vi "Query Frequency Mode.vi"(8 "error in (no error)":errorcluster, 11 "VISA resource name":refnum<visa-resource-name>) -> (0 "error out":errorcluster, 2 "Frequency Mode":T1(ring), 3 "VISA resource name out":refnum<visa-resource-name>)   [LabVIEW 2017, in "Agilent PSG MXG Series.lvlib"]
uses:
  Agilent PSG MXG Series.lvlib
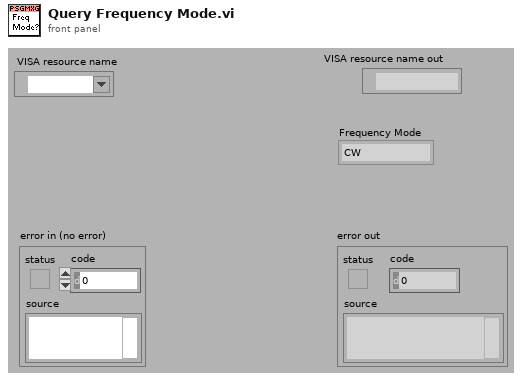
[diagram p1: front panel]
types:
  T1 = enum16{"CW", "Fixed", "Stepped Sweep", "List Sweep"}
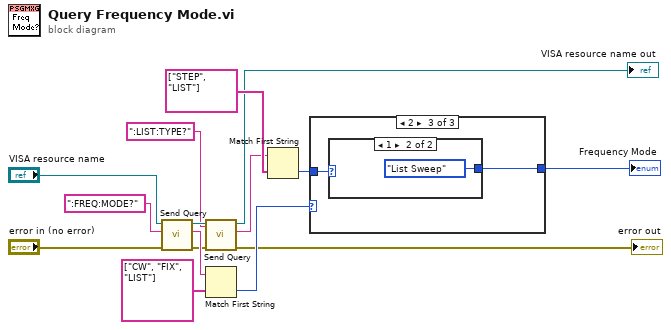
[diagram p0: block diagram]
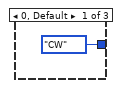
[diagram p2: hidden frame]
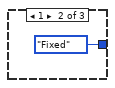
[diagram p3: hidden frame]
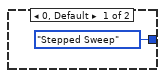
[diagram p4: hidden frame]
diagram:
  n1 = call "Send Query.vi"("error in (no error)"="error in (no error)", "write buffer"=":FREQ:MODE?", "VISA resource name"="VISA resource name") -> ("error out"=w7:errorcluster, "read buffer"=w10:string, "VISA resource name out"=w9:refnum<visa-resource-name>)  [unwired: 6 out]
  n2 = call "Send Query.vi"("error in (no error)"=w7, "write buffer"=":LIST:TYPE?", "VISA resource name"=w9) -> ("error out"=→"error out":errorcluster, "read buffer"=w6:string, "VISA resource name out"=→"VISA resource name out":refnum<visa-resource-name>)  [unwired: 6 out]
  n3 = Match First String(2:string[] ["CW", "FIX", "LIST"], 3:w10) -> (0:w5:i32)  [unwired: 1 out]
  n4 = Match First String(2:string[] ["STEP", "LIST"], 3:w6) -> (0:w3:i32)  [unwired: 1 out]
  n5 = case shown="2" w5 {
    tunnel: [T1."CW" ("Frequency Mode") T1."Fixed" ("Frequency Mode") w18] -> w4
    tunnel: w3 -> [_ _ w19]
    frame 0, Default {
    }
    frame 1 {
    }
    frame 2 {
      n6 = case shown="1" w19 {
        tunnel: [T1."Stepped Sweep" ("Frequency Mode") T1."List Sweep" ("Frequency Mode")] -> w18
        frame 0, Default {
        }
        frame 1 {
        }
      }
    }
  }
  "Frequency Mode" <- w4
